vi "passing data through while loops.vi"() -> ()   [LabVIEW 2018]
uses:
  <vilib>/DAQmx/read.llb/DAQmx Read (Analog 1D DBL NChan 1Samp).vi
  <vilib>/DAQmx/miscellaneous.llb/DAQmx Fill In Error Info.vi
panel:
  out "element 4":dbl
  out "Array 2":dbl[](array[numeric])
  out "element 3":dbl
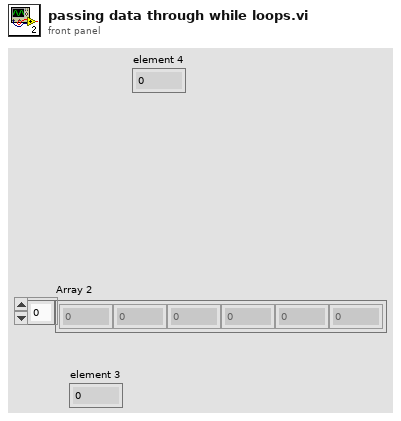
[diagram p1: front panel]
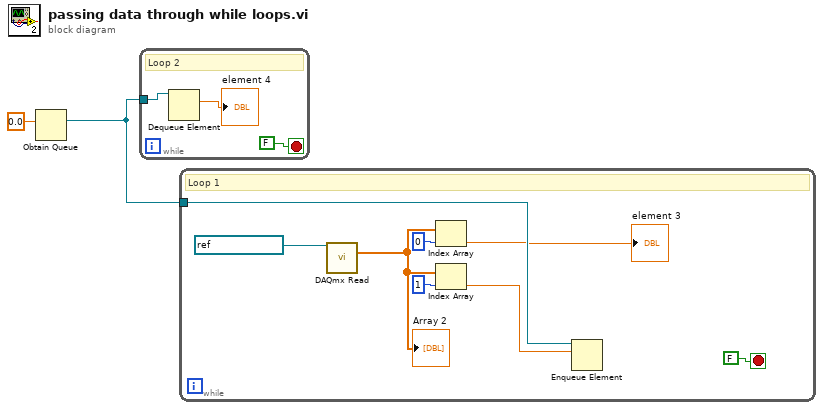
[diagram p0: block diagram]
diagram:
  n1 = Obtain Queue(element data type=0.0) -> (queue out=w1:refnum<queue>)  [unwired: 4 in, 2 out]
  n2 = while {
    tunnel: w1 -> [w5]
    stop <- FALSE stop-if-true
    # "Loop 2"
    n3 = Dequeue Element(queue=w5) -> (element=→"element 4":dbl)  [unwired: 2 in, 3 out]
  }
  n4 = while {
    tunnel: w1 -> [w13]
    stop <- FALSE stop-if-true
    # "Loop 1"
    n5 = call-poly <vilib>:"DAQmx Read.vi"("task/channels in"=refnum<k21> "1_4_2_7_6_5") -> ("data"=w9:dbl[])  [unwired: 12 in, 2 out]
    "Array 2" <- w9
    n6 = Index Array(array=w9, index=0) -> (element=→"element 3":dbl)
    n7 = Index Array(array=w9, index=1) -> (element=w7:dbl)
    n8 = Enqueue Element(queue=w13, element=w7) -> ()  [unwired: 2 in, 3 out]
  }
